vi "tcs_salCommander_enable.vi"(8 "error in (no error)":errorcluster) -> (0 "error out":errorcluster, 3 "function return":i32)   [LabVIEW 2016, in "SALLV_tcs.lvlib"]
doc: "int tcs_shm_salCommander_enableLV();"
uses:
  SALLV_tcs.lvlib
  SALLV_tcs.so
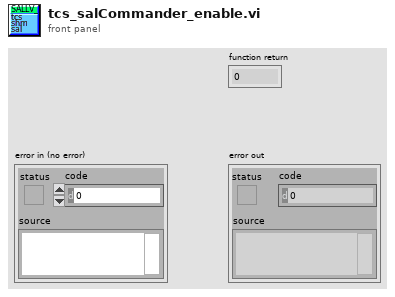
[diagram p1: front panel]
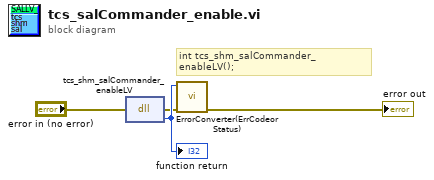
[diagram p0: block diagram]
diagram:
  # "int tcs_shm_salCommander_enableLV();"
  n1 = dll-call lib="home/andres/Desktop/SALLV_tcs/SALLV_tcs.*" fn="tcs_shm_salCommander_enableLV"(error in="error in (no error)") -> (error out=w2:errorcluster, w4:i32)  [unwired: 2 in, 1 out]
  "function return" <- w4
  n2 = call "ErrorConverter(ErrCodeorStatus).vi"("error in (no error)"=w2, "error code"=w4) -> ("error out"=→"error out":errorcluster)  [unwired: 9 in]
